vi "ROV Control via UDP Protocole.vi"() -> ()   [LabVIEW 2012]
uses:
  <vilib>/Utility/inputDevices.llb/closeJoystick.vi
  <vilib>/Utility/inputDevices.llb/joystickAcquire.vi
panel:
  out "Y-Axis 5":dbl
  out "direction info":T1
  out "Current\nCase":T2(ring)=enum."B5"
  out "String":string="0000 C"
  out "Y-Axis":string caption="Result"
  out "Y-Axis 2":dbl
  out "X-Axis":dbl
  out "X-Axis 2":string caption="Result"
  in  "stop":bool
  in  "device index":i32
  in  "Enum":T2(ring)=enum."B5"
  out "axis info":T3
  out "button info":T4
  in  "stop 2":bool
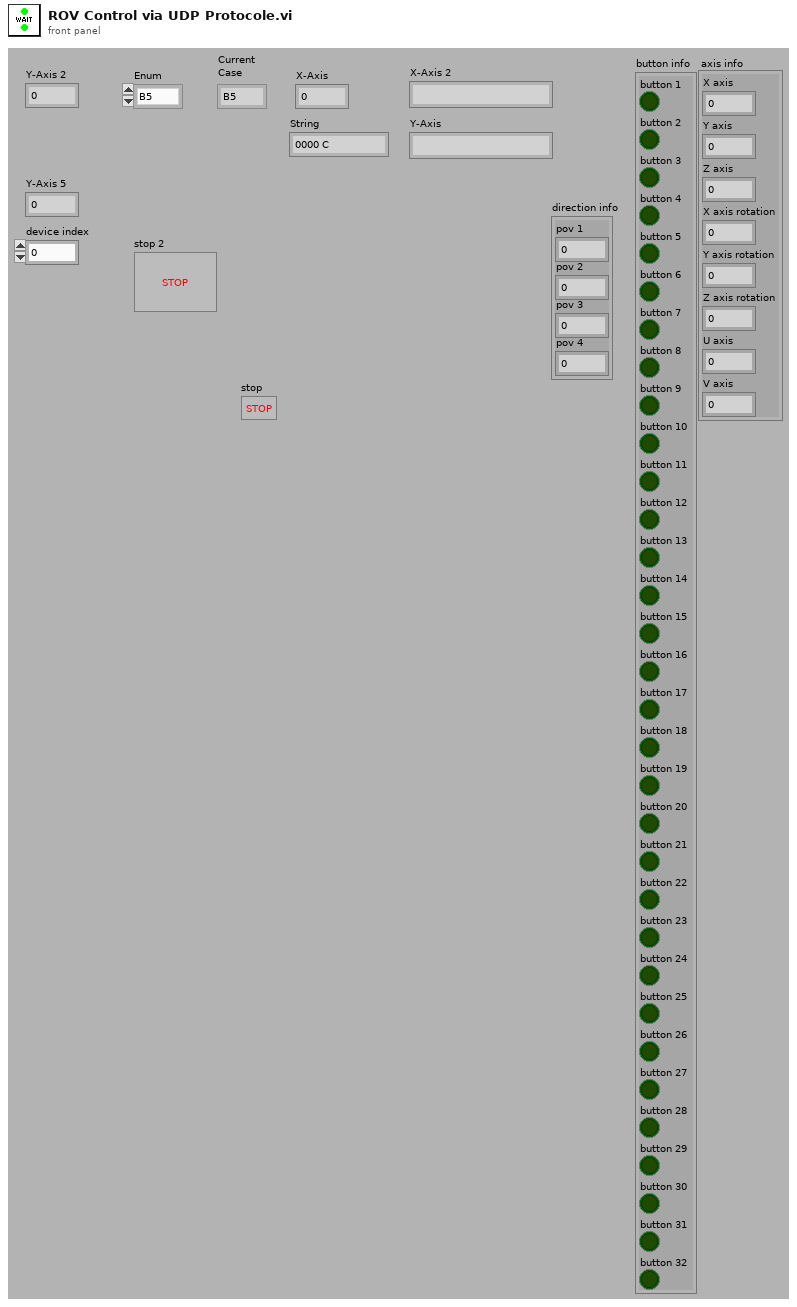
[diagram p1: front panel]
types:
  T1 = cluster{"pov 1":i32, "pov 2":i32, "pov 3":i32, "pov 4":i32}
  T2 = enum16{"", "B5", "B8", "B9", "B10", "B11", "B12", "B6", "B7", "B4", "B3", "B2", "Null", "X axis", "Y axis"}
  T3 = cluster{"X axis":i32, "Y axis":i32, "Z axis":i32, "X axis rotation":i32, "Y axis rotation":i32, "Z axis rotation":i32, "U axis":i32, "V axis":i32}
  T4 = cluster{"button 1":bool, "button 2":bool, "button 3":bool, "button 4":bool, "button 5":bool, "button 6":bool, "button 7":bool, "button 8":bool, "button 9":bool, "button 10":bool, "button 11":bool, "button 12":bool, "button 13":bool, "button 14":bool, "button 15":bool, "button 16":bool, "button 17":bool, "button 18":bool, "button 19":bool, "button 20":bool, "button 21":bool, "button 22":bool, "button 23":bool, "button 24":bool, "button 25":bool, "button 26":bool, "button 27":bool, "button 28":bool, "button 29":bool, "button 30":bool, "button 31":bool, "button 32":bool}
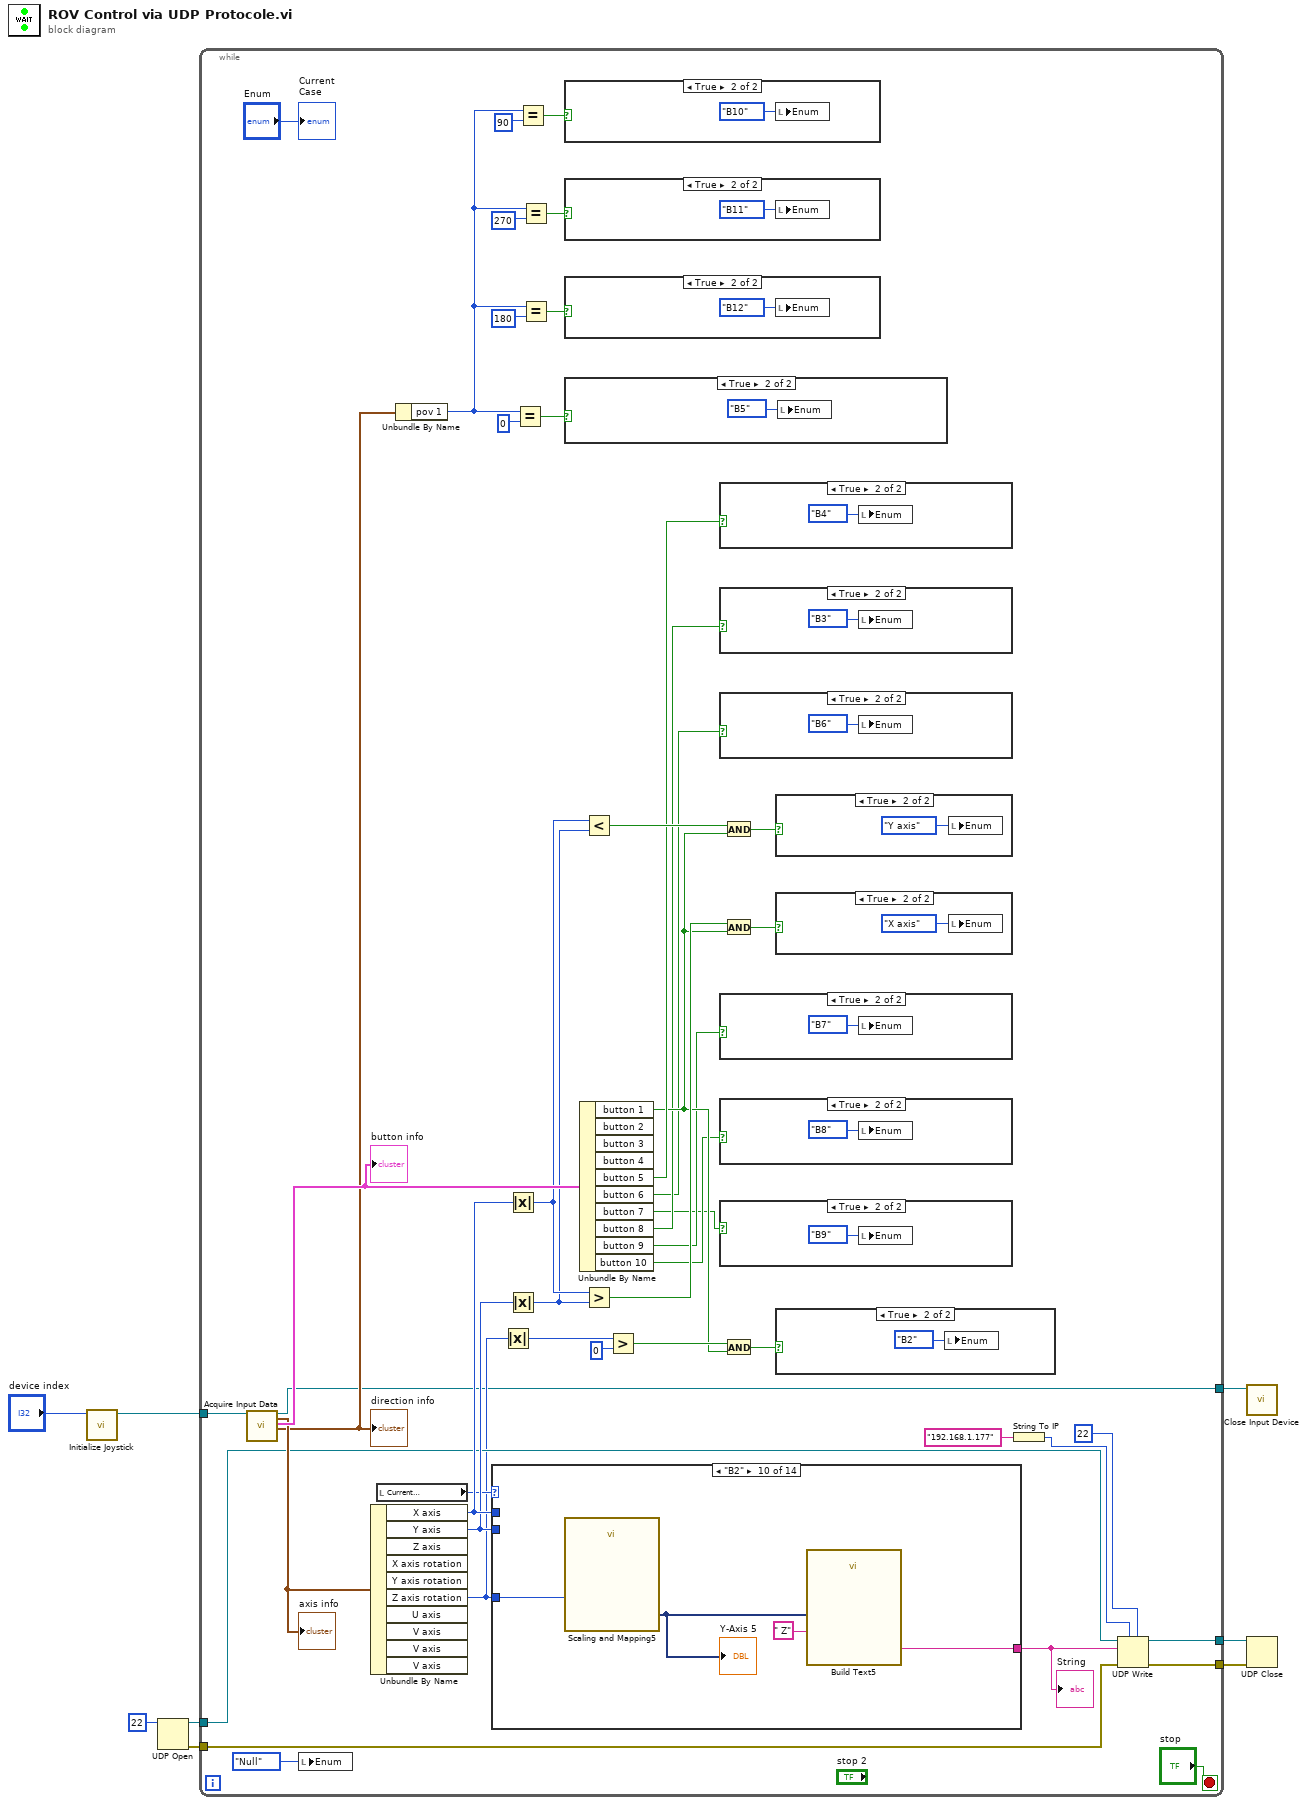
[diagram p0: block diagram]
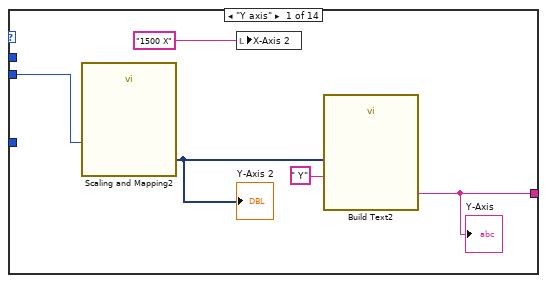
[diagram p14: hidden frame]
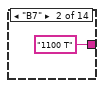
[diagram p15: hidden frame]
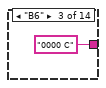
[diagram p16: hidden frame]
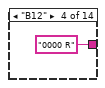
[diagram p17: hidden frame]
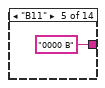
[diagram p18: hidden frame]
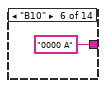
[diagram p19: hidden frame]
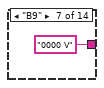
[diagram p20: hidden frame]
diagram:
  n1 = call <vilib>:"Initialize Joystick.vi"("device index"="device index") -> ("device ID"=w7:refnum<k1>)  [unwired: 9 in, 1 out]
  n2 = UDP Open(11:u16 22 ("port")) -> (port=w3:refnum<k16>, 0:w2:errorcluster)  [unwired: 4 in, 1 out]
  n3 = while {
    tunnel: w7 -> [w50]
    tunnel: [w39] -> w5
    tunnel: [w38] -> w4
    tunnel: w3 -> [w37]
    tunnel: w2 -> [w36]
    tunnel: [w16] -> w1
    stop <- "stop" stop-if-true
    n4 = call-poly <vilib>:"Acquire Input Data.vi"("device ID"=w50) -> ("device ID"=w16:refnum<k1>, "axis info"=w53:T3, "button info"=w54:T4, "direction info"=w32:T1)  [unwired: 14 in, 1 out]
    "button info" <- w54
    "axis info" <- w53
    "direction info" <- w32
    n5 = local write "Enum"(T2."Null" ("Enum")) -> ()
    n6 = Unbundle By Name(w53) -> ("X axis"=w44:i32, "Y axis"=w43:i32, "Z axis rotation"=w21:i32)  [unwired: 7 out]
    n7 = local read "Current\nCase"() -> (w26:T2)
    n8 = Unbundle By Name(w32) -> ("pov 1"=w27:i32)
    n9 = case shown="\"B2\"" w26 {
      tunnel: w44 -> [_ _ _ _ _ _ _ _ _ _ _ _ _ w90]
      tunnel: w43 -> [w69 _ _ _ _ _ _ _ _ _ _ _ _ _]
      tunnel: [w67 "1100 T" "0000 C" "0000 R" "0000 B" "0000 A" "0000 V" "1900 M" "0000 L" w80 "0000 Q" "0000 O" "1500 N" ("Result") w88] -> w35
      tunnel: w21 -> [_ _ _ _ _ _ _ _ _ w81 _ _ _ _]
      frame "Y axis" {
        n10 = call "Scaling and Mapping2"("Signals"=w69) -> ("Scaled Signals"=w71:dynamicdata)  [unwired: 9 in, 1 out]
        "Y-Axis 2" <- w71
        n11 = local write "X-Axis 2"("1500 X") -> ()
        n12 = call "Build Text2"("value"=w71, "Y"=" Y" ("X")) -> ("Result"=w67:string)  [unwired: 12 in, 1 out]
        "Y-Axis" <- w67
      }
      frame "B7" {
      }
      frame "B6" {
      }
      frame "B12" {
      }
      frame "B11" {
      }
      frame "B10" {
      }
      frame "B9" {
      }
      frame "B8" {
      }
      frame "B5" {
      }
      frame "B2" {
        n13 = call "Scaling and Mapping5"("Signals"=w81) -> ("Scaled Signals"=w83:dynamicdata)  [unwired: 9 in, 1 out]
        "Y-Axis 5" <- w83
        n14 = call "Build Text5"("value"=w83, "Y"=" Z" ("X")) -> ("Result"=w80:string)  [unwired: 12 in, 1 out]
      }
      frame "B3" {
      }
      frame "B4" {
      }
      frame "Null", Default {
      }
      frame "X axis" {
        n15 = call "Scaling and Mapping"("Signals"=w90) -> ("Scaled Signals"=w91:dynamicdata)  [unwired: 9 in, 1 out]
        "X-Axis" <- w91
        n16 = local write "Y-Axis"("1500 Y") -> ()
        n17 = call "Build Text"("value"=w91, "X"=" X") -> ("Result"=w88:string)  [unwired: 12 in, 1 out]
        "X-Axis 2" <- w88
      }
    }
    "String" <- w35
    n18 = Absolute Value(x=w21) -> (abs(x)=w20:i32)
    n19 = Absolute Value(x=w44) -> (abs(x)=w49:i32)
    n20 = Absolute Value(x=w43) -> (abs(x)=w48:i32)
    n21 = Equal?(x=w27, y=0) -> (x = y?=w25:bool)
    n22 = Equal?(x=w27, y=90) -> (x = y?=w23:bool)
    n23 = Equal?(x=w27, y=270) -> (x = y?=w22:bool)
    n24 = Equal?(x=w27, y=180) -> (x = y?=w24:bool)
    n25 = case shown="True" w23 {
      frame False {
      }
      frame True {
        n26 = local write "Enum"(T2."B10" ("Enum")) -> ()
      }
    }
    n27 = case shown="True" w22 {
      frame False {
      }
      frame True {
        n28 = local write "Enum"(T2."B11" ("Enum")) -> ()
      }
    }
    n29 = case shown="True" w24 {
      frame False {
      }
      frame True {
        n30 = local write "Enum"(T2."B12" ("Enum")) -> ()
      }
    }
    n31 = case shown="True" w25 {
      frame False {
      }
      frame True {
        n32 = local write "Enum"(T2."B5" ("Enum")) -> ()
      }
    }
    n33 = Unbundle By Name(w54) -> ("button 1"=w15:bool, "button 5"=w34:bool, "button 6"=w10:bool, "button 7"=w9:bool, "button 8"=w11:bool, "button 9"=w13:bool, "button 10"=w12:bool)  [unwired: 3 out]
    n34 = Less?(x=w49, y=w48) -> (x < y?=w47:bool)
    n35 = Greater?(x=w49, y=w48) -> (0:w52:bool)
    n36 = Greater?(x=w20, y=0) -> (0:w18:bool)
    n37 = case shown="True" w34 {
      frame False {
      }
      frame True {
        n38 = local write "Enum"(T2."B4" ("Enum")) -> ()
      }
    }
    n39 = case shown="True" w11 {
      frame False {
      }
      frame True {
        n40 = local write "Enum"(T2."B3" ("Enum")) -> ()
      }
    }
    n41 = case shown="True" w10 {
      frame False {
      }
      frame True {
        n42 = local write "Enum"(T2."B6" ("Enum")) -> ()
      }
    }
    n43 = case shown="True" w13 {
      frame False {
      }
      frame True {
        n44 = local write "Enum"(T2."B7" ("Enum")) -> ()
      }
    }
    n45 = case shown="True" w12 {
      frame False {
      }
      frame True {
        n46 = local write "Enum"(T2."B8" ("Enum")) -> ()
      }
    }
    n47 = case shown="True" w9 {
      frame False {
      }
      frame True {
        n48 = local write "Enum"(T2."B9" ("Enum")) -> ()
      }
    }
    n49 = And(x=w47, y=w15) -> (x .and. y?=w46:bool)
    n50 = And(x=w52, y=w15) -> (x .and. y?=w51:bool)
    n51 = And(x=w18, y=w15) -> (x .and. y?=w14:bool)
    n52 = case shown="True" w46 {
      frame False {
      }
      frame True {
        n53 = local write "Enum"(T2."Y axis" ("Enum")) -> ()
      }
    }
    n54 = case shown="True" w51 {
      frame False {
      }
      frame True {
        n55 = local write "Enum"(T2."X axis" ("Enum")) -> ()
      }
    }
    n56 = case shown="True" w14 {
      frame False {
      }
      frame True {
        n57 = local write "Enum"(T2."B2" ("Enum")) -> ()
      }
    }
    n58 = String To IP(1:"192.168.1.177" ("name")) -> (0:w41:u32)
    n59 = UDP Write(address=w41, port or service name=u16 22, connection ID=w37, data in=w35, 8:w36) -> (error out=w38:errorcluster, 3:w39:refnum<k16>)  [unwired: 1 in]
    "Current\nCase" <- "Enum"
  }
  n60 = call-poly <vilib>:"Close Input Device.vi"("device ID"=w1) -> ()  [unwired: 9 in, 1 out]
  n61 = UDP Close(connection ID=w5, 8:w4) -> ()  [unwired: 2 out]
